vi "Backup Path.vi"(8 "error in (no error)":errorcluster) -> (0 "error out":errorcluster, 3 "pg_backup.txt path":path)   [LabVIEW 2019, in "LV-Data.PGSQL.lvclass"]
uses:
  LV-Data.PGSQL.lvclass
  <vilib>/Utility/sysdir.llb/System Directory Type.ctl
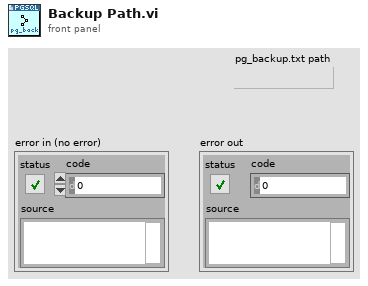
[diagram p1: front panel]
types:
  T1 = typedef "System Directory Type.ctl" = i32
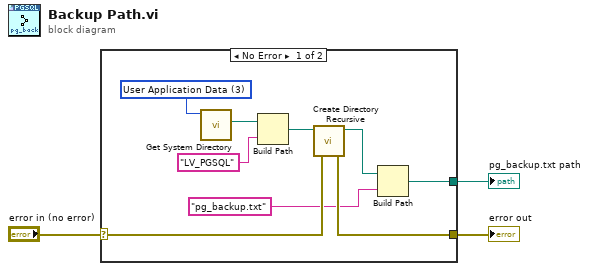
[diagram p0: block diagram]
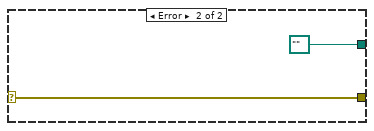
[diagram p2: hidden frame]
diagram:
  n1 = case shown="No Error" "error in (no error)" {
    selector: "error in (no error)" -> [w9 w14]
    tunnel: [w8 w14] -> w3
    tunnel: [w7 path "" ("appended path")] -> w1
    frame No Error {
      w12 = T1 3 items=["User Home"=0, "User Desktop"=1, "User Documents"=2, "User Application Data"=3, "User Preferences"=4, "User Temporary"=5, "Public Documents"=6, "Public Application Data"=7, "Public Preferences"=8, "Public Cache"=13, "System Core Libraries"=9, "System Installed Libraries"=10, "Application Files"=11, "Boot Volume Root"=12] ("system directory type")
      n2 = call <vilib>:"Get System Directory.vi"("system directory type"=w12) -> ("system directory"=w11:path)  [unwired: 10 in]
      n3 = Build Path(base path=w11, name or relative path="LV_PGSQL") -> (appended path=w6:path)
      n4 = call <vilib>:"Create Directory Recursive.vi"("error in (no error)"=w9, "directory"=w6) -> ("error out"=w8:errorcluster, "directory copy"=w4:path)  [unwired: 3 in, 1 out]
      n5 = Build Path(base path=w4, name or relative path="pg_backup.txt") -> (appended path=w7:path)
    }
    frame Error {
    }
  }
  "error out" <- w3
  "pg_backup.txt path" <- w1
